vi "Read.vi"(8 "error in (no error)":errorcluster, 11 "Mouse Controller in":refnum<class "Mouse.lvclass">) -> (0 "error out":errorcluster, 1 "Velocity out":dbl, 2 "Direction out":cluster{dbl, dbl}, 4 "Stop?":bool, 5 "Boost?":bool)   [LabVIEW 2024, in "Mouse.lvclass"]
doc: "MIT Licence\nCopyright (c) 2024 David Grollier"
uses:
  Mouse.lvclass
  Input Device.lvclass/Input Device.ctl
  Mouse.lvclass/Mouse.ctl
  <vilib>/Utility/inputDevices.llb/mouseAcquire.vi
  Utils/Utils.lvlib
  Input Device.lvclass
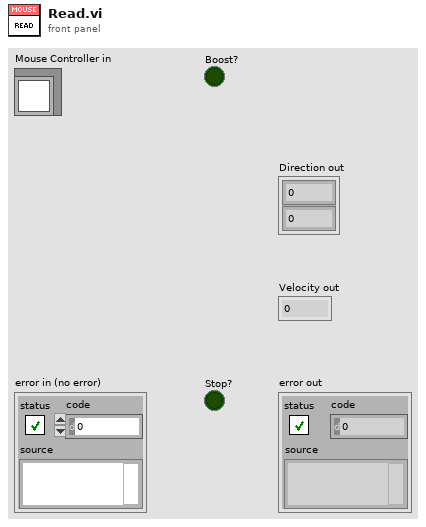
[diagram p1: front panel]
types:
  T1 = typedef "LVRectTypeDef.ctl" = cluster{"Left":i16, "Top":i16, "Right":i16, "Bottom":i16}
  T2 = cluster{"Horizontal":i32, "Vertical":i32, "Scrolling":i32}
  T3 = cluster{"Stop Event Registration Refnum out":refnum<event-registration>, "Event Registration Refnum":refnum<event-registration>}
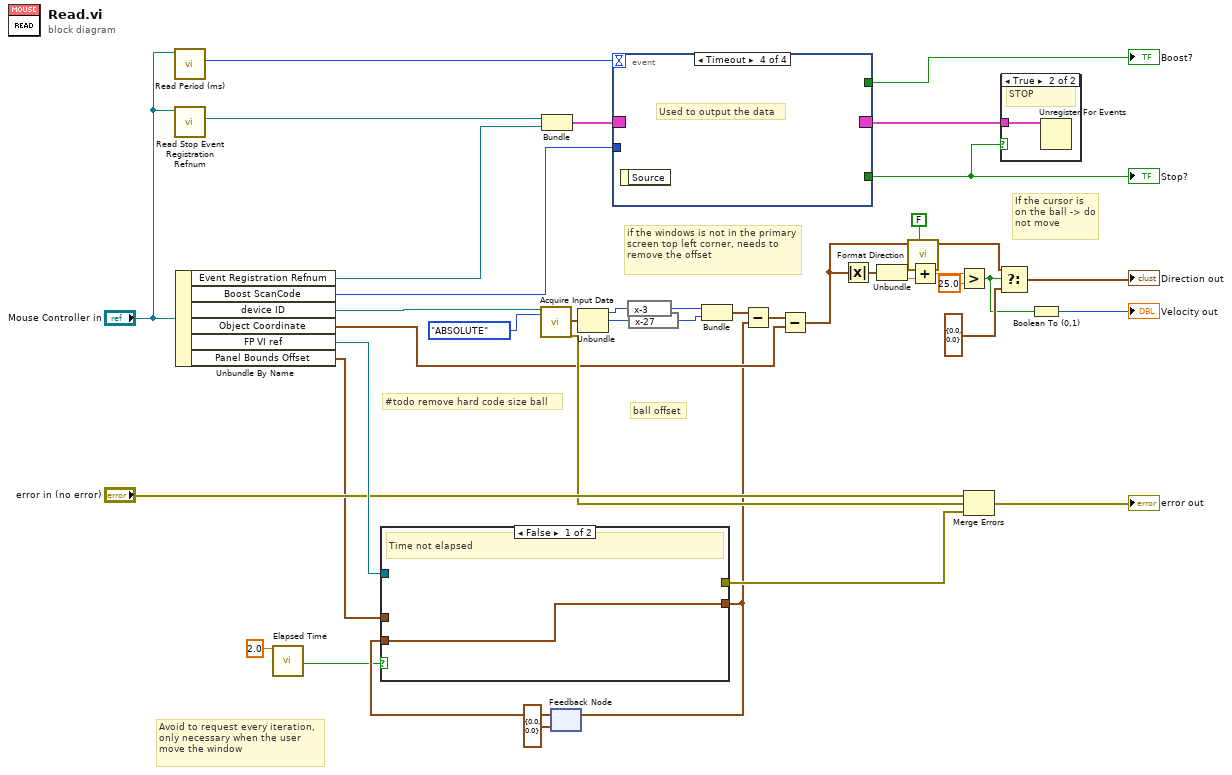
[diagram p0: block diagram]
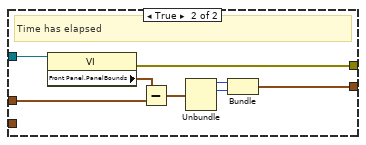
[diagram p2: hidden frame]
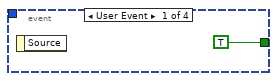
[diagram p4: hidden frame]
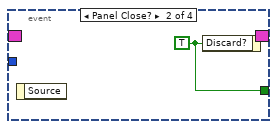
[diagram p5: hidden frame]
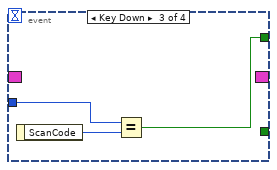
[diagram p6: hidden frame]
diagram:
  # "#todo remove hard code size ball"
  # "ball offset"
  # "Avoid to request every iteration, only necessary when the user move the window"
  # "if the windows is not in the primary screen top left corner, needs to remove the offset"
  # "If the cursor is on the ball -> do not move"
  n1 = call "Read Period (ms).vi"("Input Device in"="Mouse Controller in") -> ("Period (ms)"=w17:i64)  [unwired: 10 in]
  n2 = call "Read Stop Event Registration Refnum.vi"("Input Device in"="Mouse Controller in") -> ("Stop Event Registration Refnum out"=w25:refnum<event-registration>)  [unwired: 10 in]
  n3 = Unbundle By Name("Mouse Controller in") -> ("Event Registration Refnum"=w24:refnum<event-registration>, "Boost ScanCode"=w20:i16, "device ID"=w26:refnum<k1>, "Object Coordinate"=w7:cluster{"Horizontal":i32, "Vertical":i32}, "FP VI ref"=w14:refnum<vi>, "Panel Bounds Offset"=w1:T1)
  n4 = call "Elapsed Time"("Time Target (s)"=2.0) -> ("Time has Elapsed"=w2:bool)  [unwired: 11 in, 7 out]
  n5 = call-poly <vilib>:"Acquire Input Data.vi"("device ID"=w26, "key mode"=enum16{"RELATIVE", "ABSOLUTE"}."ABSOLUTE") -> ("axis info"=w36:T2, "error out"=w11:errorcluster)  [unwired: 14 in, 2 out]
  n6 = Bundle("Stop Event Registration Refnum out"=w25, "Event Registration Refnum"=w24) -> (w23:T3)  [unwired: 1 in]
  n7 = feedback #1(cluster{dbl, dbl} {0.0, 0.0}) -> (w4:cluster{"Left":dbl, "Top":dbl})
  n8 = case shown="False" w2 {
    tunnel: w14 -> [_ w51]
    tunnel: [_ w47] -> w10
    tunnel: [w43 w48] -> w5
    tunnel: w4 -> [w43 _]
    tunnel: w1 -> [_ w45]
    frame False {
      # "Time not elapsed"
    }
    frame True {
      # "Time has elapsed"
      n9 = property class="VI"(reference=w51) -> (error out=w47:errorcluster, "Front Panel.PanelBounds"=w46:T1)  [unwired: 1 in, 1 out]
      n10 = Subtract(x=w46, y=w45) -> (x-y=w44:T1)
      n11 = Unbundle(w44) -> ("Left"=w50:i16, "Top"=w49:i16)  [unwired: 2 out]
      n12 = Bundle("Left"=w50, "Top"=w49) -> (w48:cluster{"Left":i16, "Top":i16})  [unwired: 1 in]
    }
  }
  n13 = feedback-in #1(w5) -> ()
  n14 = Unbundle(w36) -> ("Horizontal"=w37:i32, "Vertical"=w38:i32)  [unwired: 1 out]
  n15 = event shown="[3] Timeout" {
    selector: w23 -> [_ _ _ _]
    dyn-events: [_ _ _ _] -> w42
    timeout: w17 -> [_ _ _ _]
    tunnel: [TRUE w53 _ _] -> w21
    tunnel: w20 -> [_ _ w55 _]
    tunnel: [_ _ w54 _] -> w19
    event User Event {
      n16 = event-data() -> ()  [unwired: 1 in, 1 out]
    }
    event Panel Close? {
      w53 = TRUE ("Discard?")
      n17 = event-data() -> ()  [unwired: 1 in, 1 out]
      n18 = event-data("Discard?"=w53) -> ()  [unwired: 1 in, 1 out]
    }
    event Key Down {
      n19 = event-data() -> ("ScanCode"=w56:i16)  [unwired: 1 in]
      n20 = Equal?(x=w55, y=w56) -> (x = y?=w54:bool)
    }
    event Timeout {
      # "Used to output the data"
      n21 = event-data() -> ()  [unwired: 1 in, 1 out]
    }
  }
  "Boost?" <- w19
  "Stop?" <- w21
  n22 = expression code="x-3"(w37) -> (w41:i32)
  n23 = expression code="x-27"(w38) -> (w40:i32)
  n24 = Bundle("Horizontal"=w41, "Vertical"=w40) -> (w39:cluster{"Horizontal":i32, "Vertical":i32})  [unwired: 1 in]
  n25 = Subtract(x=w39, y=w5) -> (x-y=w9:cluster{dbl, dbl})
  n26 = Subtract(x=w9, y=w7) -> (x-y=w8:cluster{dbl, dbl})
  n27 = Absolute Value(x=w8) -> (abs(x)=w33:cluster{dbl, dbl})
  n28 = Unbundle(w33) -> (w28:dbl, w29:dbl)
  n29 = call "Format Direction.vi"("Xbox Controller (T)"=FALSE ("Analog Stick? (T)"), "Direction in"=w8) -> ("Formated Direction out"=w31:cluster{dbl, dbl})  [unwired: 9 in]
  n30 = Add(x=w28, y=w29) -> (x+y=w34:dbl)
  n31 = Greater?(x=w34, y=25.0) -> (0:w22:bool)
  n32 = Merge Errors("error in (no error)", w11, w10) -> (→"error out":errorcluster)
  n33 = Select(t=w31, s=w22, f=cluster{dbl, dbl} {0.0, 0.0} ("t")) -> (s? t:f=→"Direction out":cluster{dbl, dbl})
  n34 = case shown="True" w21 {
    tunnel: w42 -> [_ w57]
    frame False {
      # "No Stop"
    }
    frame True {
      # "STOP"
      n35 = Unregister For Events(event registration refnum=w57) -> ()  [unwired: 1 in, 1 out]
    }
  }
  n36 = Boolean To (0,1)(Boolean=w22) -> (0, 1=→"Velocity out":i16)
